vi "Create Project.vi"(6 "Authorization":T1[](array[typedef]), 8 "error in (no error)":errorcluster, 10 "Description":string, 11 "Name":string) -> (0 "error out":errorcluster, 2 "gid":string)   [LabVIEW 2016]
uses:
  <vilib>/addons/_JKI.lib/REST Client/classes/REST Client/HTTP Header.ctl
  <vilib>/addons/_JKI.lib/REST Client/classes/REST Client/REST Client.lvclass
  <vilib>/addons/_JKI.lib/Serialization/JSON/JKI JSON Serialization.lvlib
panel:
  out "Response body":string
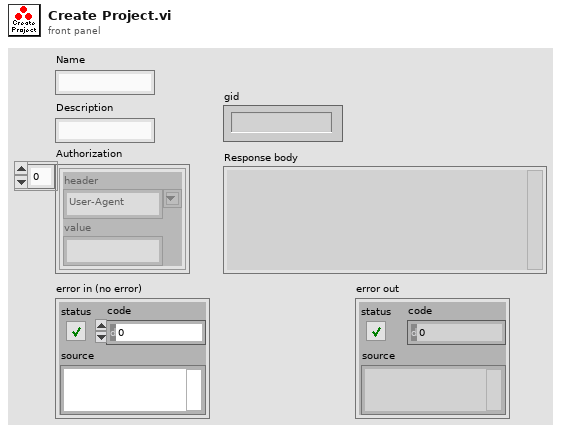
[diagram p1: front panel]
types:
  T1 = typedef "REST Client.lvlib/REST Client.lvclass/HTTP Header.ctl" = cluster{"header":string, "value":string}
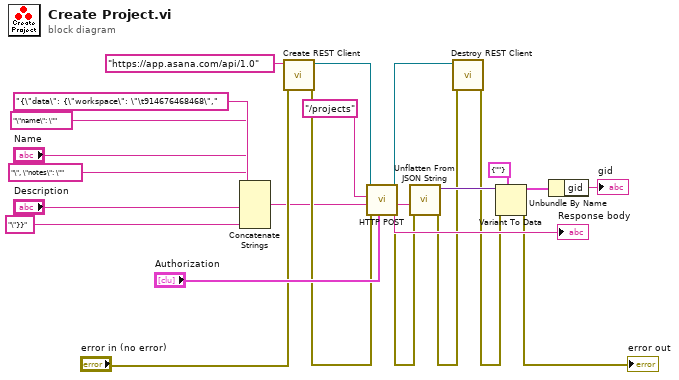
[diagram p0: block diagram]
diagram:
  n1 = Concatenate Strings("{\"data\": {\"workspace\": \"\t914676468468\",", "\"name\": \"" ("string"), "Name", "\", \"notes\": \"" ("string"), "Description", "\"}}" ("string")) -> (w16:string)
  n2 = call <vilib>:"Create REST Client.vi"("error in (no error)"="error in (no error)", "Base URL"="https://app.asana.com/api/1.0") -> ("error out"=w17:errorcluster, "REST Client out"=w21:refnum<class "REST Client.lvclass">)  [unwired: 8 in]
  n3 = call-dynamic "HTTP POST.vi"("request specific headers"="Authorization", "error in (no error)"=w17, "Request body"=w16, "Path"="/projects", "REST Client in"=w21) -> ("error out"=w13:errorcluster, "Response body"=w14:string, "REST Client out"=w20:refnum<class "REST Client.lvclass">)  [unwired: 1 in, 3 out]
  "Response body" <- w14
  n4 = call <vilib>:"Unflatten From JSON String.vi"("error in (no error)"=w13, "JSON String"=w14) -> ("error out"=w12:errorcluster, "Variant"=w15:variant)  [unwired: 8 in]
  n5 = call-dynamic "Destroy REST Client.vi"("error in (no error)"=w12, "REST Client in"=w20) -> ("error out"=w11:errorcluster)  [unwired: 9 in]
  n6 = Variant To Data(error in=w11, type=cluster{"gid":string} {"gid"=""}, Variant=w15) -> (data=w8:cluster{"gid":string}, error out=→"error out":errorcluster)
  n7 = Unbundle By Name(w8) -> ("gid"=→"gid":string)
